vi "Open Session.vi"(8 "error in (no error)":errorcluster, 10 "port number or service name (3363)":u16=3363, 11 "machine name (\"\":  local reference)":string="localhost") -> (0 "error out":errorcluster, 3 "ApplicationAPI out":refnum<class "TemplateAPI.lvclass">)   [LabVIEW 2018, in "TemplateAPI.lvclass"]
uses:
  TemplateAPI.lvclass
  C:/Users/Phalanx/Documents/LabVIEW-Application-API-Template/Classes/AppControlAPI/AppControlAPI.lvclass
  AppControlAPI/AppControlAPI.lvclass
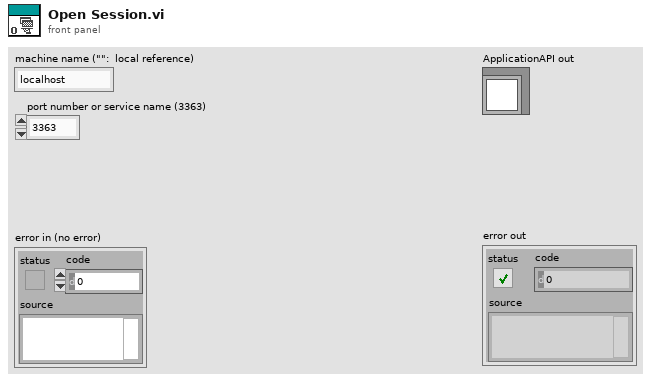
[diagram p1: front panel]
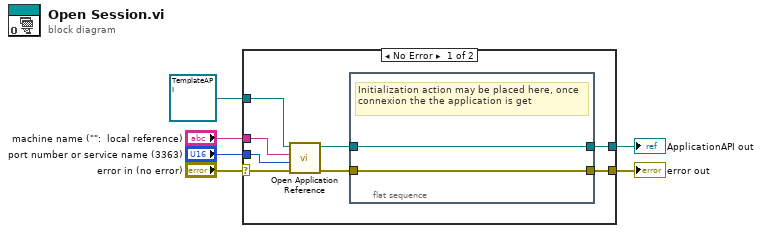
[diagram p0: block diagram]
diagram:
  n1 = case shown="No Error" "error in (no error)" {
    selector: "error in (no error)" -> [w9 w18]
    tunnel: [w14 w18] -> w5
    tunnel: [w13 w17] -> w2
    tunnel: refnum<class "TemplateAPI.lvclass"> refnum ("ApplicationAPI out") -> [w12 w17]
    tunnel: "machine name (\"\":  local reference)" -> [w11 _]
    tunnel: "port number or service name (3363)" -> [w10 _]
    frame No Error {
      n2 = call "Open Application Reference.vi"("error in (no error)"=w9, "port number or service name (3363)"=w10, "machine name (\"localhost\")"=w11, "App Control API in"=w12) -> ("error out"=w7:errorcluster, "App Control API out"=w8:refnum<class "TemplateAPI.lvclass">)  [unwired: 6 in]
      n3 = flat-sequence {
        tunnel: w7 -> [w16]
        tunnel: [w16] -> w14
        tunnel: w8 -> [w15]
        tunnel: [w15] -> w13
        frame #0 {
          # "Initialization action may be placed here, once connexion the the application is get"
        }
      }
    }
    frame Error {
    }
  }
  "error out" <- w5
  "ApplicationAPI out" <- w2
